vi "Draw Gradient.vi"(9 "draw options":T1={"Outer Border Color"=0, "Inner Border Color"=6316128, "Outer Gradient Color"=2565927, "Inner Gradient Color"=16860, "Compass North Pointer Color"=16711680, "Compass Pointer Color 1"=13355429, "Compass Pointer Color 2"=14934973, "Direction Pointer Color"=16765184, "Text Box Outline Color"=13355429, "Text Box Background Color"=14934973, "Scale Color"=16448250, "Text Color"=0, "Draw Gradient"=TRUE, "Draw Rose"=TRUE, "Simple Scale"=TRUE, "Draw Text"=FALSE, "Font Name"="Helvetica", "Angle Units"=enum."Degrees"}, 10 "draw area cache in":T3, 11 "picture in":picture) -> (3 "picture out":picture)   [LabVIEW 2017, in "NI_Robotics_Compass Picture.lvlib"]
uses:
  <vilib>/robotics/Controls/Compass Indicator/Compass Picture/NI_Robotics_Compass Picture.lvlib
  <vilib>/robotics/Controls/Compass Indicator/Compass Picture/Draw Area State.ctl
  <vilib>/Utility/miscctls.llb/LVBoundsTypeDef.ctl
  <vilib>/robotics/Controls/Compass Indicator/Compass Picture/Draw Options.ctl
  <vilib>/robotics/Controls/Utilities/Angle Units.ctl
  <vilib>/robotics/Controls/Utilities/NI_Robotics_Control Utilities.lvlib
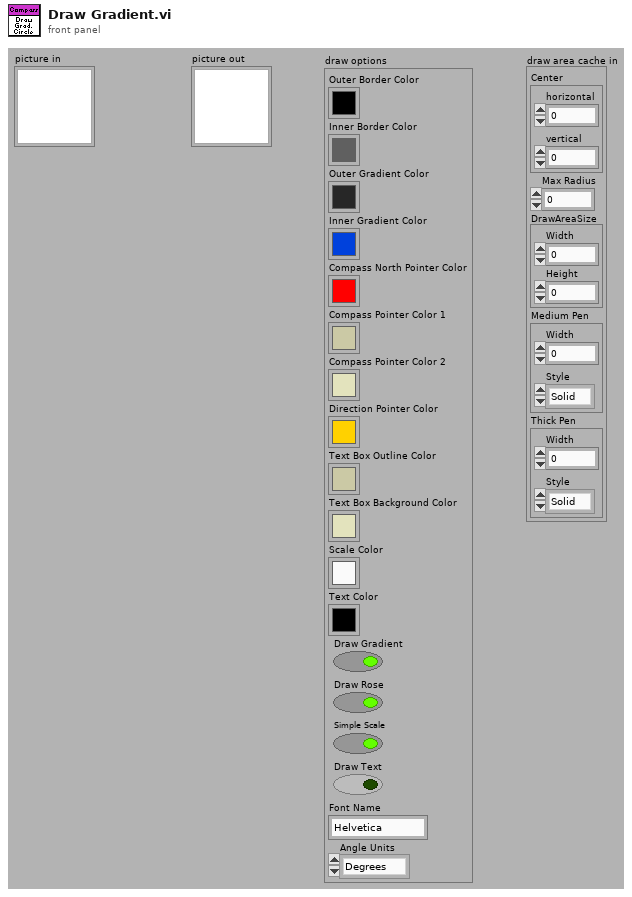
[diagram p1: front panel]
types:
  T1 = typedef "NI_Robotics_Compass Picture.lvlib/Draw Options.ctl" = cluster{"Outer Border Color":u32, "Inner Border Color":u32, "Outer Gradient Color":u32, "Inner Gradient Color":u32, "Compass North Pointer Color":u32, "Compass Pointer Color 1":u32, "Compass Pointer Color 2":u32, "Direction Pointer Color":u32, "Text Box Outline Color":u32, "Text Box Background Color":u32, "Scale Color":u32, "Text Color":u32, "Draw Gradient":bool, "Draw Rose":bool, "Simple Scale":bool, "Draw Text":bool, "Font Name":string, "Angle Units":T2}
  T2 = typedef "NI_Robotics_Control Utilities.lvlib/Angle Units.ctl" = enum16{"Radians", "Degrees"}
  T3 = typedef "NI_Robotics_Compass Picture.lvlib/Draw Area State.ctl" = cluster{"Center":cluster{"horizontal":i16, "vertical":i16}, "Max Radius":dbl, "DrawAreaSize":T4, "Medium Pen":cluster{"Width":u16, "Style":enum32{"Solid", "Dash", "Dot", "DashDot", "DashDotDot"}}, "Thick Pen":cluster{"Width":u16, "Style":enum32{"Solid", "Dash", "Dot", "DashDot", "DashDotDot"}}}
  T4 = typedef "LVBoundsTypeDef.ctl" = cluster{"Width":u32, "Height":u32}
  T5 = cluster{"Width":u16, "Style":enum32{"Solid", "Dash", "Dot", "DashDot", "DashDotDot"}}
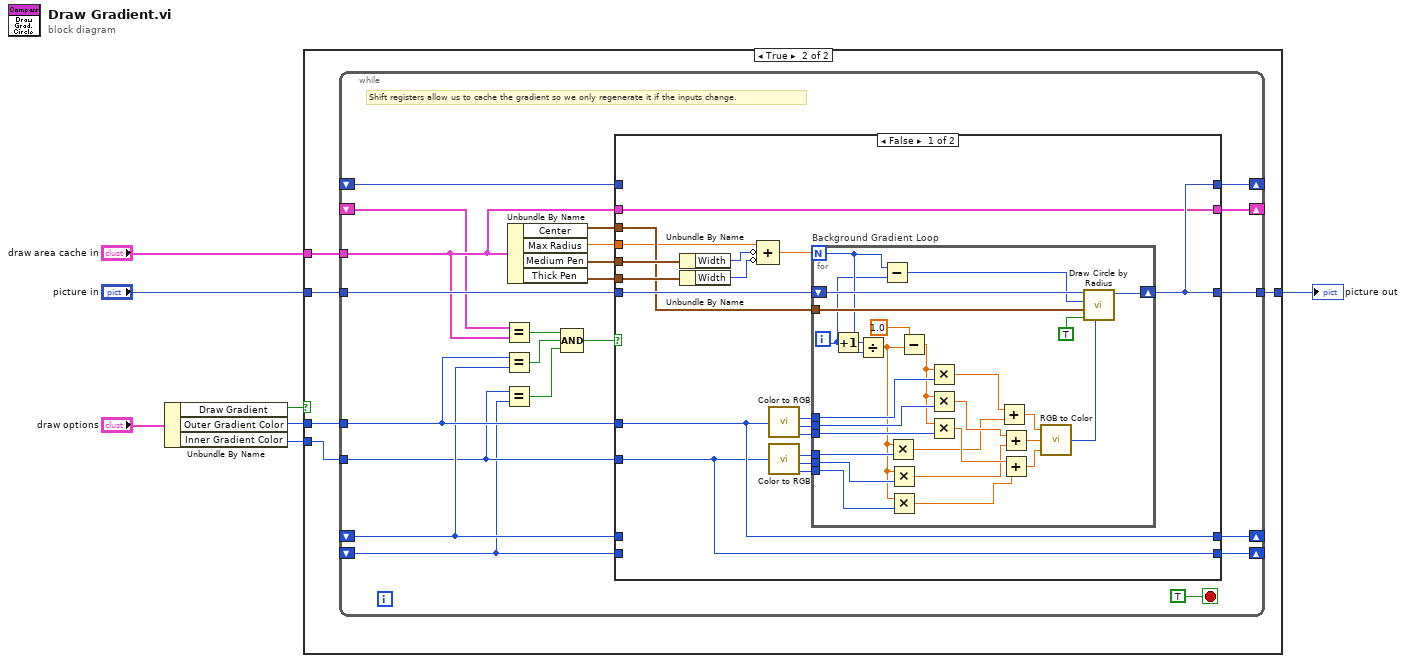
[diagram p0: block diagram]
diagram:
  n1 = Unbundle By Name("draw options") -> ("Draw Gradient"=w1:bool, "Outer Gradient Color"=w2:u32, "Inner Gradient Color"=w3:u32)
  n2 = case shown="True" w1 {
    tunnel: [w8 w13] -> w7
    tunnel: "picture in" -> [w8 w12]
    tunnel: "draw area cache in" -> [_ w11]
    tunnel: w3 -> [_ w10]
    tunnel: w2 -> [_ w9]
    frame False {
    }
    frame True {
      n3 = while {
        tunnel: [w35] -> w13
        tunnel: w10 -> [w22]
        tunnel: w9 -> [w24]
        tunnel: w12 -> [w34]
        tunnel: w11 -> [w18]
        shift-right: [w28] -> _
        shift-left: _ -> [w23]
        shift-right: [w27] -> _
        shift-left: _ -> [w21]
        shift-right: [w26] -> _
        shift-left: _ -> [w25]
        shift-right: [w17] -> _
        shift-left: _ -> [w16]
        stop <- TRUE stop-if-true
        # "Shift registers allow us to cache the gradient so we only regenerate it if the inputs change."
        n4 = Equal?(x=w16, y=w18) -> (x = y?=w15:bool)
        n5 = Equal?(x=w24, y=w23) -> (x = y?=w20:bool)
        n6 = Equal?(x=w22, y=w21) -> (x = y?=w19:bool)
        n7 = Unbundle By Name(w18) -> ("Center"=w33:cluster{"horizontal":i16, "vertical":i16}, "Max Radius"=w32:dbl, "Medium Pen"=w31:T5, "Thick Pen"=w30:T5)
        n8 = Compound Arithmetic op=AND(w15, w20, w19) -> (w14:bool)
        n9 = case shown="False" w14 {
          tunnel: [w44 w84] -> w35
          tunnel: w32 -> [w42 _]
          tunnel: w30 -> [w53 _]
          tunnel: w31 -> [w52 _]
          tunnel: w22 -> [w37 _]
          tunnel: w24 -> [w38 _]
          tunnel: w34 -> [w45 _]
          tunnel: w33 -> [w43 _]
          tunnel: [w44 w84] -> w26
          tunnel: w25 -> [_ w84]
          tunnel: [w38 w83] -> w28
          tunnel: [w37 w82] -> w27
          tunnel: w21 -> [_ w82]
          tunnel: w23 -> [_ w83]
          tunnel: w18 -> [w36 w81]
          tunnel: [w36 w81] -> w17
          frame False {
            n10 = Unbundle By Name(w52) -> ("Width"=w40:u16)
            n11 = Unbundle By Name(w53) -> ("Width"=w41:u16)
            n12 = Compound Arithmetic op=ADD(w42, invert w40, invert w41) -> (w39:dbl)
            n13 = call <vilib>:"Color to RGB.vi"("Color"=w38) -> ("R"=w46:u8, "G"=w47:u8, "B"=w48:u8)  [unwired: 1 out]
            n14 = call <vilib>:"Color to RGB.vi"("Color"=w37) -> ("R"=w49:u8, "G"=w50:u8, "B"=w51:u8)  [unwired: 1 out]
            n15 = for "Background Gradient Loop" {
              N: w39 -> [w60]
              shift-right: [w79] -> w44
              shift-left: w45 -> [w80]
              tunnel: w46 -> [w74]
              tunnel: w47 -> [w73]
              tunnel: w48 -> [w72]
              tunnel: w49 -> [w77]
              tunnel: w50 -> [w76]
              tunnel: w51 -> [w75]
              tunnel: w43 -> [w62]
              i -> [w59]
              n16 = Increment(x=w59) -> (x+1=w57:i32)
              n17 = Divide(x=w57, y=w60) -> (x/y=w56:dbl)
              n18 = Subtract(x=w60, y=w59) -> (x-y=w61:i32)
              n19 = Multiply(x=w56, y=w77) -> (x*y=w68:dbl)
              n20 = Multiply(x=w56, y=w76) -> (x*y=w67:dbl)
              n21 = Multiply(x=w56, y=w75) -> (x*y=w66:dbl)
              n22 = Subtract(x=1.0, y=w56) -> (x-y=w55:dbl)
              n23 = Multiply(x=w55, y=w74) -> (x*y=w71:dbl)
              n24 = Multiply(x=w55, y=w73) -> (x*y=w70:dbl)
              n25 = Multiply(x=w55, y=w72) -> (x*y=w69:dbl)
              n26 = Add(x=w71, y=w68) -> (x+y=w65:dbl)
              n27 = Add(x=w70, y=w67) -> (x+y=w64:dbl)
              n28 = Add(x=w69, y=w66) -> (x+y=w63:dbl)
              n29 = call <vilib>:"RGB to Color.vi"("B"=w63, "G"=w64, "R"=w65) -> ("Color"=w58:u32)
              n30 = call <vilib>:"Draw Circle by Radius.vi"("color(black)"=w58, "fill?(F)"=TRUE, "pixel center"=w62, "radius"=w61, "picture"=w80) -> ("new picture"=w79:picture)  [unwired: 6 in]
            }
          }
          frame True {
          }
        }
      }
    }
  }
  "picture out" <- w7
